vi "Queue Reference (library variable).vi"() -> ()   [LabVIEW 2023, in "Error Manager.lvlib" / "New Error Window.lvlib" / "MHL Queue.lvlib"]
uses:
  MHL Queue.lvlib
  Message (cluster).ctl
  Command (enum).ctl
panel:
  in  "Queue Reference":refnum<queue>
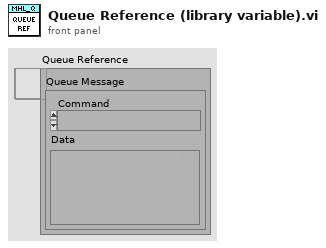
[diagram p1: front panel]
diagram:
